vi "simple RX 2955 sync.vi"() -> ()   [LabVIEW 2021]
uses:
  <vilib>/userdefined/High Color/nirio_resource_hc.ctl
  states.ctl
  <vilib>/Analysis/4window.llb/windowTd.ctl
  <vilib>/Analysis/coordinate.llb/Angle Range (Degree).ctl
  <vilib>/Analysis/coordinate.llb/Angle Units.ctl
  <vilib>/Analysis/coordinate.llb/Wrap Angle (scalar).vi
  <instrlib>/_niInstr/DSP/v1/FPGA/Public/Sub VIs/Data Conversion/U32 to IQ - 1 spc - S18.1.vi
  <vilib>/measure/maspectr.llb/FFT Spectrum (Mag-Phase) for 1 Chan (CDB).vi
  <vilib>/FPGAPlugInAG/USRP 2945; 2955/niLvFpga_Open_USRP 2945; 2955.vi
  <vilib>/rvi/interface/common/dynamic/niFpgaDynamicAddResources.vi
  <vilib>/FPGAPlugInAG/Dynamic/niLvFpga_Download_Dynamic.vi
  <vilib>/FPGAPlugInAG/Dynamic/niLvFpga_Run_Dynamic.vi
  <vilib>/rvi/interface/common/niFpgaWaitOnOcc.vi
  <vilib>/Utility/error.llb/Error Cluster From Error Code.vi
  <vilib>/rvi/errors/niLvFpgaAdjustHostInterfaceError.vi
  <vilib>/rvi/interface/nirviOpenFPGA/nirviOpenFPGA.xnode
  FPGA Bitfiles/Streaming 2955 simple.lvbitx
  <vilib>/rvi/interface/nirviMethod/nirviMethod.xnode
  <vilib>/rvi/interface/nirviReadWriteControl/nirviReadWriteControl.xnode
  <instrlib>/niUsrpRio/Config/v1/Host/niUsrpRio Config v1 Host.lvlib
  <vilib>/Analysis/NI_AAL_Angle.lvlib
  <instrlib>/_niInstr/DSP/v1/FPGA/niInstr DSP v1 FPGA.lvlib
  <vilib>/Analysis/NI_AALPro.lvlib
  <vilib>/measure/NI_MAPro.lvlib
  <vilib>/rvi/errors/niLvFpgaMergeErrorWithErrorCode.vi
  <vilib>/rvi/interface/Simulation/niFpgaSimulationCallBeginRW.vi
  <vilib>/FPGAPlugInAG/Dynamic/niLvFpga_ConfigureFifo_Dynamic.vi
  NiFpgaLv.dll
  <vilib>/FPGAPlugInAG/Dynamic/niLvFpga_ReadFifo_Dynamic.vi
panel:
  in  "resource name":T1="USRP_2955"
  in  "computing load":dbl(slide) scale=0.0..20.0
  in  "max queue":i32=20
  out "FPGA lost sampels":u32=262858
  out "dt":dbl=2e-07
  out "delta phase (deg)":dbl[](array[numeric])=[0.0, -114.69647545281569, -168.47745794220134, 21.231862090137405]
  out "scop":dbl[][](graph)
  out "spectrum":cluster{"f0":dbl, "df":dbl, "magnitude":dbl[]}[](graph)
  in  "Number of Elements":u32=2048 step=1024
  in  "reset":bool
  in  "cal phase (deg)":dbl[](array[numeric])=[0.0, 0.0, 0.0, 0.0]
  in  "output sample rate":dbl=5000000.0 format="%#_6pHz"
  in  "frequency shift":dbl=5000000.0 format="%#_6pHz"
  in  "Rx. frequency":dbl=500000000.0 format="%#_6pHz"
  in  "gain":dbl=50.0 min=0.0 max=90.0 step=1.0 format="%#_6pdB"
  # "device"
  # "data out"
  # "Rx params"
  # "RF params"
  # "DSP params"
  # "computing"
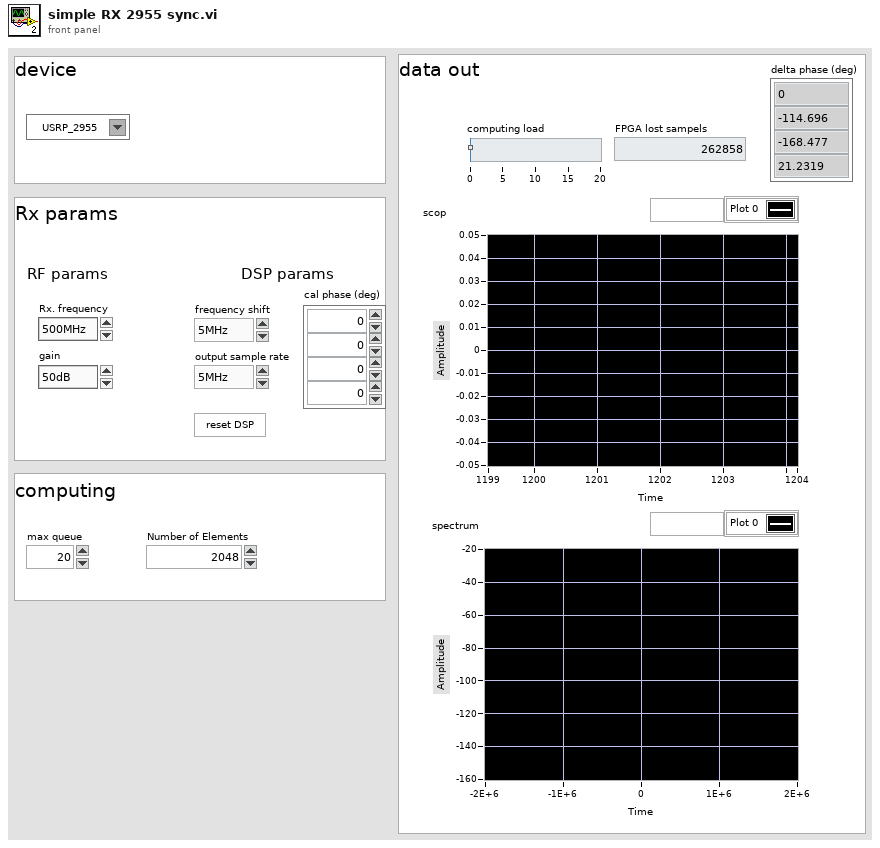
[diagram p1: front panel]
types:
  T1 = typedef "nirio_resource_hc.ctl" = tag
  T2 = typedef "states.ctl" = enum16{"ini", "set basic", "update DSP", "close sesion", "read", "wait"}
  T3 = enum16{"ini", "set basic", "update DSP", "close sesion"}
  T4 = cluster{"daughterboard 0 lo configuration":enum16{"Independent", "Import", "Shared and Export", "Reimport", "Shared"}, "daughterboard 1 lo configuration":enum16{"Independent", "Import", "Shared and Export", "Reimport", "Shared"}}
  T5 = cluster{"output sample rate":fxp<+,48,1>, "delay":fxp<+/-,16,0>, "frequency shift":fxp<+/-,48,0>, "phase":fxp<+/-,21,0>}
  T6 = typedef "niUsrpRio Config v1 Host.lvlib/niUsrpRio Session.ctl" = cluster{"FPGA Interface":refnum<k20>, "RIO Interface Number":u32, "Data Clock Rate":u32, "FPGA Data Clock Rate":u32, "Global Settings Register Bus":T7, "Radio 0 Settings Register Bus":T7, "Radio 1 Settings Register Bus":T7, "Radio Settings Bus Semaphore":T8, "DB Queues":T9[], "Characterization Data Valid?":bool, "EEPROM Header":T10, "Device Data Header":T11, "EEPROM Characterization Header":T12, "Characterization Data":T13[], "FPGA Current Version":u32, "FPGA Oldest Compatible Version":u32, "Fixed Logic Current Version":u32, "Fixed Logic Oldest Compatible Version":u32, "FPGA Radio Settings Bus Current Version":u32, "FPGA Radio Settings Bus Oldest Compatible Version":u32, "FPGA Board Config Current Version":u32, "FPGA Board Config Oldest Compatible Version":u32, "Daughterboard Clock Rate":u32, "daughterboard configuration session handles":u64[]}
  T7 = typedef "niInstr Register Bus v0 Host.lvlib/Register Bus Session.ctl" = refnum<queue>
  T8 = typedef "Semaphore RefNum" = refnum<k1>
  T9 = typedef "niUsrpRio Config v1 Host.lvlib/DB Queue Reference.ctl" = refnum<queue>
  T10 = typedef "niUsrpRio Config v1 Host.lvlib/EEPROM Header.ctl" = cluster{"Checksum":u32, "Product Code":u16, "Hardware Current Version":u16, "Hardware Oldest Compatible Version":u16, "EEPROM Map Current Version":u16, "EEPROM Map Oldest Compatible Version":u16, "User Password":string, "Pointer to Factory Header":u32, "Pointer to User Header":u32, "Recommended Interval":u16, "Number of Reserved Bytes":i32, "Number of Daughterboards":u8, "Daughterboard IDs":u16[], "Daughterboard Serial Numbers":string[]}
  T11 = typedef "niUsrpRio Config v1 Host.lvlib/EEPROM Device Data Header.ctl" = cluster{"Checksum":u32, "Number of Channels":u8, "Number of Gain Settings":u16[], "Pointer to Characterization Data":u32[], "Number of Reserved Bytes":i32, "Number of Frequencies":u16[]}
  T12 = typedef "niUsrpRio Config v1 Host.lvlib/EEPROM Characterization Header.ctl" = cluster{"Checksum":u32, "Date":timestamp, "Temperature":sgl, "Misc. Info":string, "Pointer to Device Data Header":u32, "Number of Reserved Bytes":i32}
  T13 = typedef "niUsrpRio Config v1 Host.lvlib/Characterization Data.ctl" = cluster{"Gains[dB]":dbl[], "Frequencies [Hz]":dbl[], "IQ Imbalance Table":T14[], "Measured Gains[dB]":dbl[][]}
  T14 = typedef "niUsrpRio Config v1 Host.lvlib/IQ Imbalance.ctl" = cluster{"Gain Imbalance [linear]":dbl, "Phase Imbalance [radians]":dbl, "Offset":cdb}
  T15 = cluster{"output sample rate":fxp<+,48,1>, "delay":fxp<+/-,16,0>, "frequency shift":fxp<+/-,48,0>, "phase":fxp<+/-,21,0>}[]
  T16 = typedef "NI_AAL_Angle.lvlib/Angle Units.ctl" = i32
  T17 = typedef "NI_AAL_Angle.lvlib/Angle Range (Degree).ctl" = u16
  T18 = cluster{"dB On (F)":bool, "unwrap phase (F)":bool, "convert to degree (F)":bool}
  T19 = typedef "niInstr DSP v1 Shared.lvlib/IQ Data.ctl" = cluster{"I":fxp<+/-,18,1>, "Q":fxp<+/-,18,1>, "overflow":bool}
  T20 = typedef "NI_AALPro.lvlib/windowTd.ctl" = u32
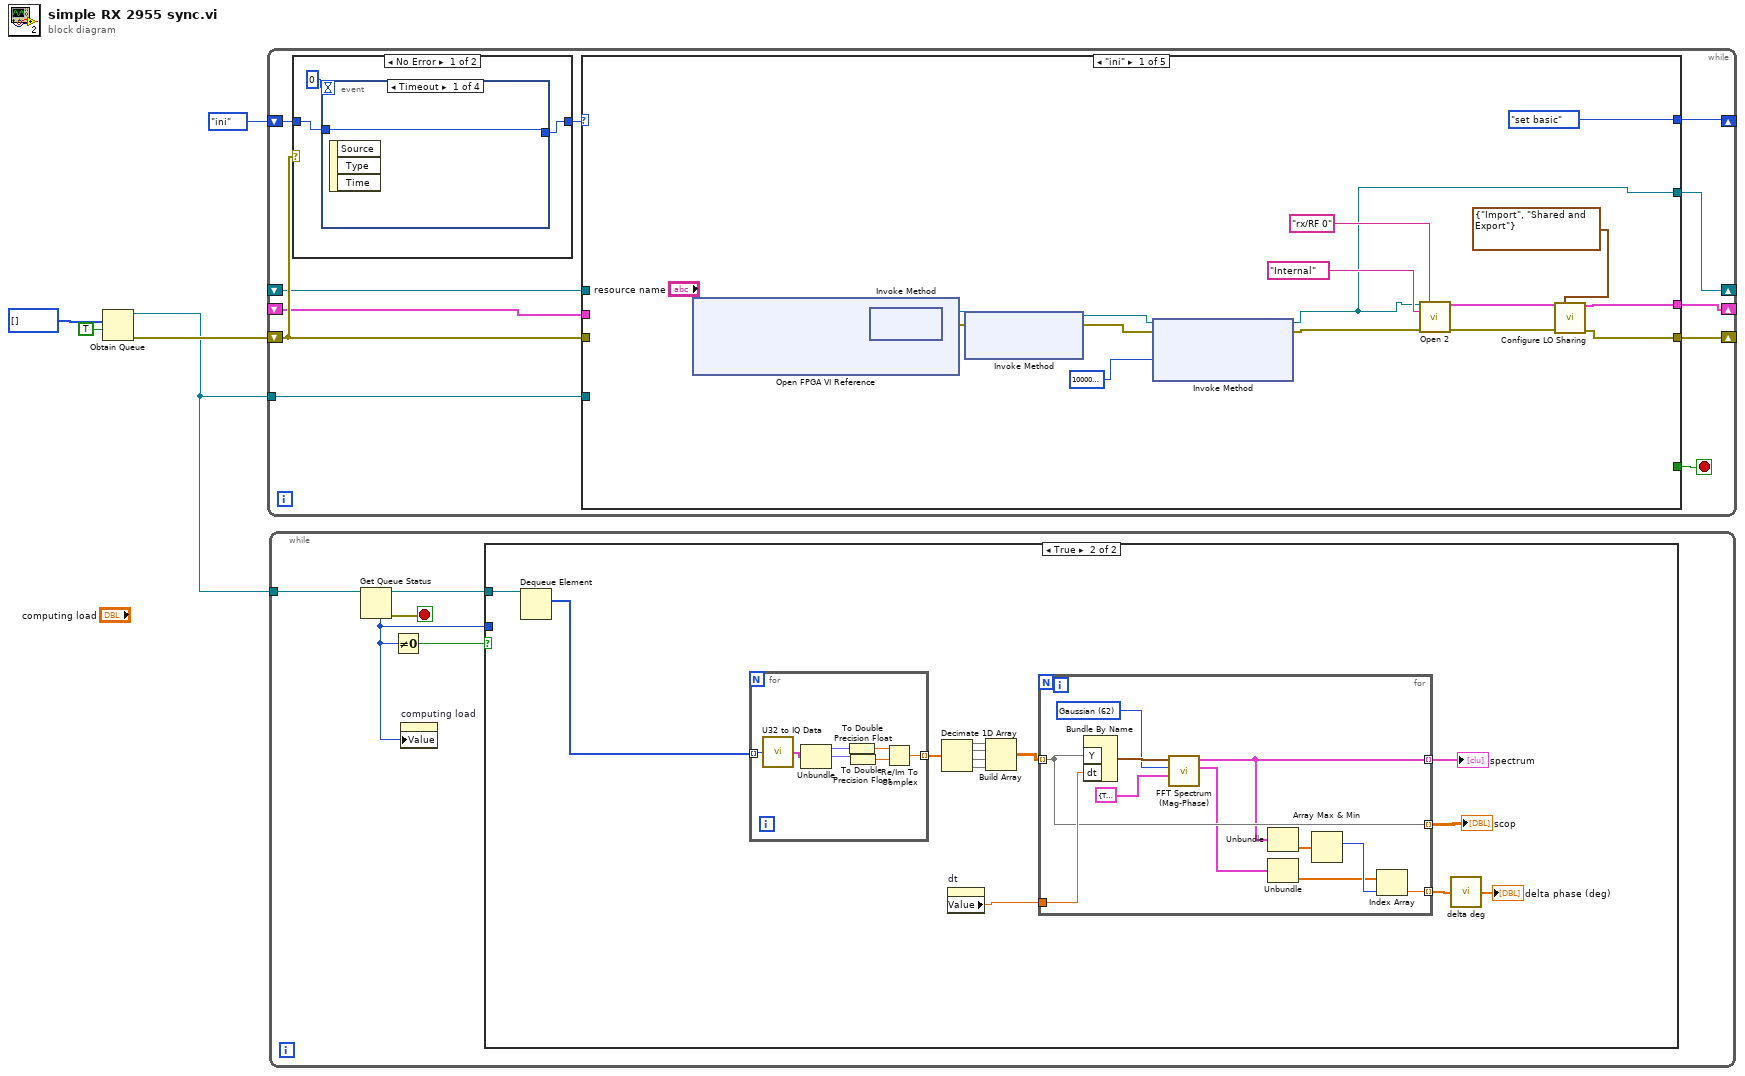
[diagram p0: block diagram]
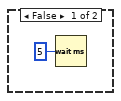
[diagram p2: hidden frame]
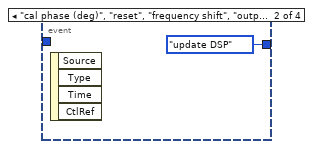
[diagram p3: hidden frame]
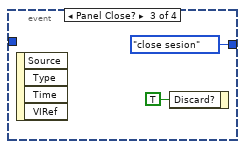
[diagram p4: hidden frame]
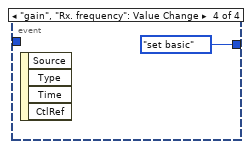
[diagram p5: hidden frame]
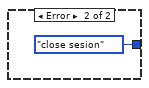
[diagram p6: hidden frame]
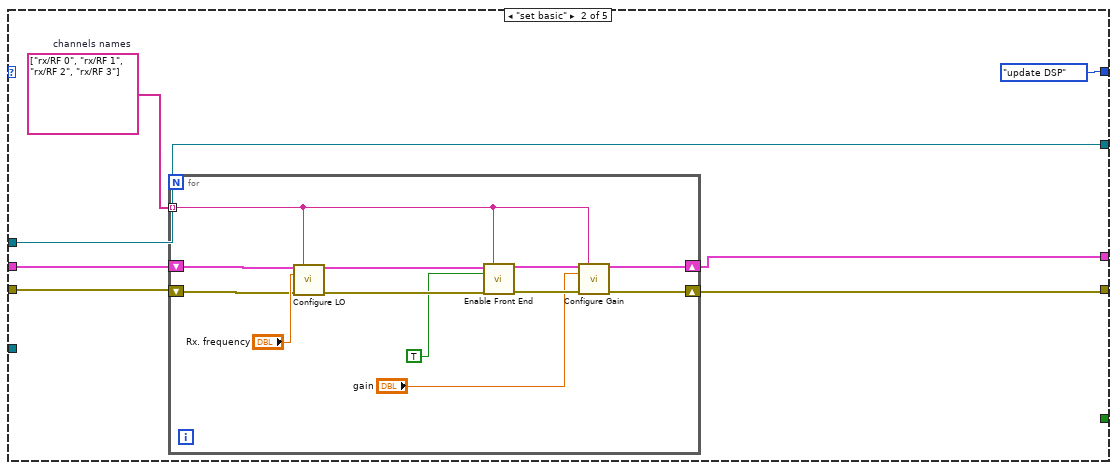
[diagram p7: hidden frame]
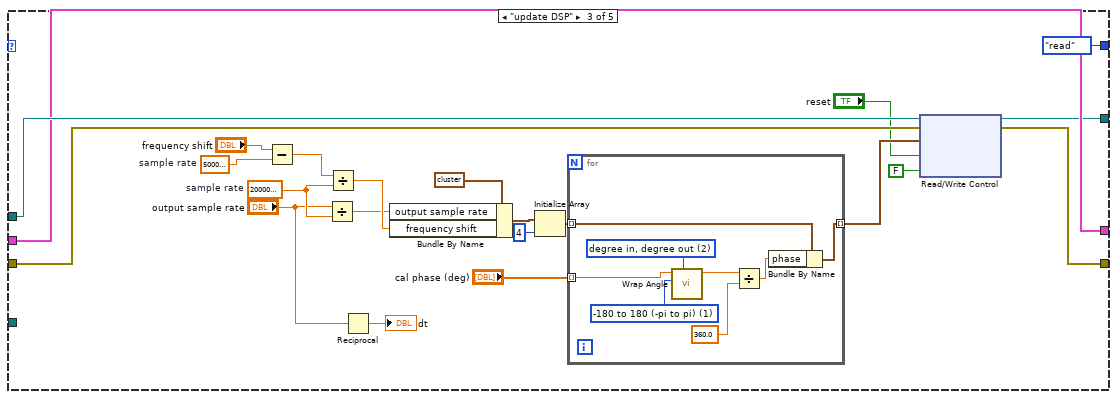
[diagram p8: hidden frame]
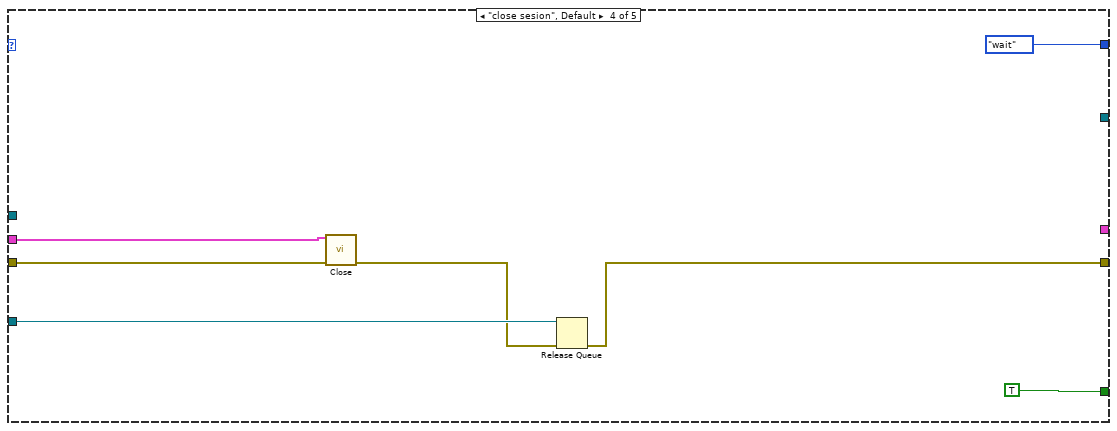
[diagram p9: hidden frame]
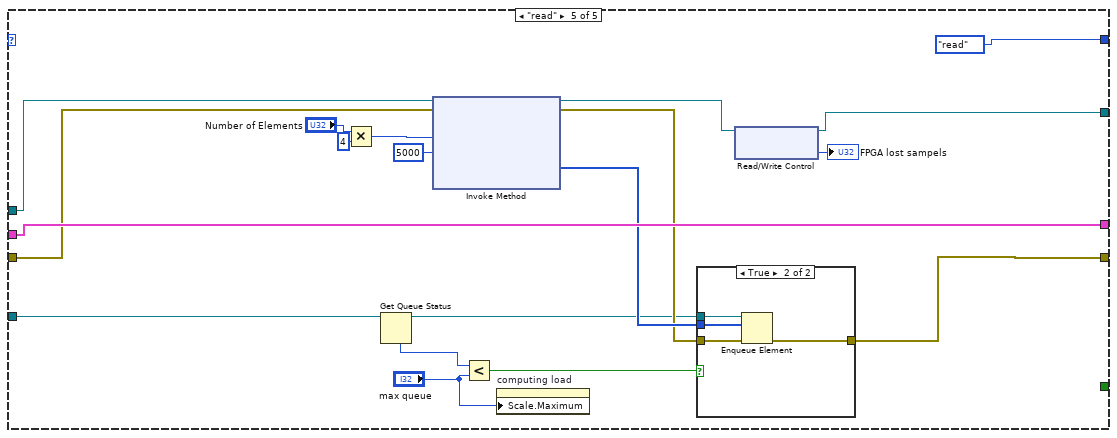
[diagram p10: hidden frame]
diagram:
  n1 = Obtain Queue(element data type=u32[] [] ("Data"), create if not found? (T)=TRUE) -> (queue out=w2:refnum<queue>, error out=w3:errorcluster)  [unwired: 3 in, 1 out]
  n2 = while {
    shift-right: [w8] -> _
    shift-left: states."ini" -> [w16]
    shift-right: [w14] -> _
    shift-left: _ -> [w9]
    shift-right: [w13] -> _
    shift-left: _ -> [w10]
    shift-right: [w12] -> _
    shift-left: w3 -> [w11]
    tunnel: w2 -> [w6]
    stop <- w7 stop-if-true
    n3 = case shown="No Error" w11 {
      tunnel: w16 -> [w18 _]
      tunnel: [w17 T3."close sesion"] -> w15
      frame No Error {
        n4 = event shown="[0] Timeout" {
          selector: _ -> [_ _ _ _]
          dyn-events: _ -> [_ _ _ _]
          timeout: 0 -> [_ _ _ _]
          tunnel: w18 -> [w20 _ _ _]
          tunnel: [w20 states."update DSP" states."close sesion" states."set basic"] -> w17
          event Timeout {
            n5 = event-data() -> ()  [unwired: 1 in, 3 out]
          }
          event "cal phase (deg)", "reset", "frequency shift", "output sample rate": Value Change {
            n6 = event-data() -> ()  [unwired: 1 in, 4 out]
          }
          event Panel Close? {
            n7 = event-data() -> ()  [unwired: 1 in, 4 out]
            n8 = event-data("Discard?"=TRUE) -> ()  [unwired: 1 in, 1 out]
          }
          event "gain", "Rx. frequency": Value Change {
            n9 = event-data() -> ()  [unwired: 1 in, 4 out]
          }
        }
      }
      frame Error {
      }
    }
    n10 = case shown="\"ini\"" w15 {
      tunnel: [w28 w48 w69 _ w105] -> w14
      tunnel: [w34 w46 w71 _ w118] -> w13
      tunnel: [w33 w45 w70 w93 w108] -> w12
      tunnel: w11 -> [_ w50 w72 w99 w111]
      tunnel: w10 -> [_ w49 w71 w98 w118]
      tunnel: w9 -> [_ w48 w73 _ w116]
      tunnel: [states."set basic" states."update DSP" states."read" states."wait" states."read"] -> w8
      tunnel: [_ _ _ TRUE _] -> w7
      tunnel: w6 -> [_ _ _ w95 w104]
      frame "ini" {
        n11 = xnode "Open FPGA VI Reference"("resource name"="resource name") -> ("FPGA VI Reference Out"=w41:refnum<k20>, "error out"=w40:errorcluster)  [unwired: 1 in]
        n12 = xnode "Invoke Method"("FPGA VI Reference In"=w41, "error in"=w40) -> ("FPGA VI Reference Out"=w43:refnum<k20>, "error out"=w42:errorcluster)
        n13 = xnode "Invoke Method"("FPGA VI Reference In"=w43, "error in"=w42) -> ("FPGA VI Reference Out"=w29:refnum<k20>, "error out"=w31:errorcluster)  [unwired: 1 in]
        n14 = xnode "Invoke Method"("FPGA VI Reference In"=w29, "error in"=w31, "Requested Depth"=u32 100000000) -> ("FPGA VI Reference Out"=w28:refnum<k20>, "error out"=w30:errorcluster)  [unwired: 1 out]
        n15 = call <instrlib>:"Open 2.vi"("fpga ref"=w28, "scope"="rx/RF 0", "Reference Frequency Source"="Internal", "error in"=w30) -> ("niUsrpRio Session (out)"=w37:T6, "error out"=w36:errorcluster)  [unwired: 10 in]
        n16 = call "Configure LO Sharing.vi"("niUsrpRio Session in"=w37, "lo config"=T4 {"daughterboard 0 lo configuration"=enum."Import", "daughterboard 1 lo configuration"=enum."Shared and Export"}, "error in"=w36) -> ("niUsrpRio Session out"=w34:T6, "error out"=w33:errorcluster)  [unwired: 11 in]
      }
      frame "set basic" {
        w47 = string[] ["rx/RF 0", "rx/RF 1", "rx/RF 2", "rx/RF 3"]  # channels names
        n17 = for {
          shift-right: [w56] -> w46
          shift-left: w49 -> [w53]
          shift-right: [w55] -> w45
          shift-left: w50 -> [w52]
          tunnel: w47 -> [w51] mode=indexing
          n18 = call <instrlib>:"Configure LO.vi"("niUsrpRio Session"=w53, "scope"=w51, "frequency"="Rx. frequency", "error in"=w52) -> ("niUsrpRio Session (out)"=w62:T6, "error out"=w61:errorcluster)  [unwired: 8 in, 2 out]
          n19 = call <instrlib>:"Enable Front End.vi"("niUsrpRio Session"=w62, "scope"=w51, "enable"=TRUE ("enable 0 2"), "error in"=w61) -> ("niUsrpRio Session (out)"=w60:T6, "error out"=w59:errorcluster)  [unwired: 10 in]
          n20 = call <instrlib>:"Configure Gain.vi"("niUsrpRio Session"=w60, "scope"=w51, "gain"="gain", "error in"=w59) -> ("niUsrpRio Session (out)"=w56:T6, "error out"=w55:errorcluster)  [unwired: 9 in, 1 out]
        }
      }
      frame "update DSP" {
        w77 = 50000000.0  # sample rate
        w80 = 200000000.0  # sample rate
        n21 = Subtract(x="frequency shift", y=w77) -> (x-y=w76:dbl)
        n22 = Divide(x="output sample rate", y=w80) -> (x/y=w79:dbl)
        n23 = Divide(x=w76, y=w80) -> (x/y=w81:dbl)
        n24 = Reciprocal(x="output sample rate") -> (1/x=→"dt":dbl)
        n25 = Bundle By Name(cluster=T5 {"output sample rate"=0.0, "delay"=0.0, "frequency shift"=0.0, "phase"=0.0} ("DSP params"), "output sample rate"=w79, "frequency shift"=w81) -> (w82:T5)
        n26 = Initialize Array(w82, 4 ("dimension size")) -> (w75:T15)
        n27 = for {
          tunnel: w75 -> [w92] mode=indexing
          tunnel: [w91] -> w68 mode=indexing
          tunnel: "cal phase (deg)" -> [w87] mode=indexing
          w85 = T16 2 items=["radian in, radian out", "radian in, degree out", "degree in, degree out", "degree in, radian out"] ("angle units")
          w88 = T17 1 items=["none", "-180 to 180 (-pi to pi)", "0 to 360 (0 to 2pi)"] ("angle range")
          n28 = call-poly <vilib>:"Wrap Angle.vi"("angle units"=w85, "angle range"=w88, "angle in"=w87) -> ("angle out"=w86:dbl)  [unwired: 7 in, 1 out]
          n29 = Divide(x=w86, y=360.0) -> (x/y=w90:dbl)
          n30 = Bundle By Name(cluster=w92, "phase"=w90) -> (w91:T5)
        }
        n31 = xnode "Read/Write Control"("FPGA VI Reference In"=w73, "error in"=w72, "DSP params"=w68, "reset"="reset", "reset"=FALSE) -> ("FPGA VI Reference Out"=w69:refnum<k20>, "error out"=w70:errorcluster)
      }
      frame "close sesion", Default {
        n32 = call <instrlib>:"Close.vi"("niUsrpRio Session"=w98, "error in"=w99) -> ("error out"=w94:errorcluster)  [unwired: 12 in, 1 out]
        n33 = Release Queue(queue=w95, error in (no error)=w94) -> (error out=w93:errorcluster)  [unwired: 1 in, 2 out]
      }
      frame "read" {
        n34 = Multiply(x="Number of Elements", y=u32 4) -> (x*y=w114:u32)
        n35 = Get Queue Status(queue=w104) -> (queue out=w103:refnum<queue>, # elements in queue=w102:i32)  [unwired: 2 in, 6 out]
        n36 = xnode "Invoke Method"("FPGA VI Reference In"=w116, "error in"=w111, "Number of Elements"=w114, "Timeout (ms)"=5000) -> ("FPGA VI Reference Out"=w107:refnum<k20>, "error out"=w109:errorcluster, "Data"=w110:u32[])  [unwired: 1 out]
        n37 = Less?(x=w102, y="max queue") -> (x < y?=w101:bool)
        n38 = property on="computing load" class="Slide (strict)"("Scale.Maximum"="max queue") -> ()  [unwired: 2 in, 2 out]
        n39 = case shown="True" w101 {
          tunnel: w110 -> [_ w123]
          tunnel: w109 -> [w119 w122]
          tunnel: [w119 w121] -> w108
          tunnel: w103 -> [_ w120]
          frame False {
          }
          frame True {
            n40 = Enqueue Element(queue=w120, element=w123, error in (no error)=w122) -> (error out=w121:errorcluster)  [unwired: 1 in, 2 out]
          }
        }
        n41 = xnode "Read/Write Control"("FPGA VI Reference In"=w107) -> ("FPGA VI Reference Out"=w105:refnum<k20>, "lost sampels"=→"FPGA lost sampels":u32)  [unwired: 1 in, 1 out]
      }
    }
  }
  n42 = while {
    tunnel: w2 -> [w128]
    stop <- w125 stop-if-true
    n43 = Get Queue Status(queue=w128) -> (queue out=w126:refnum<queue>, error out=w125:errorcluster, # elements in queue=w124:i32)  [unwired: 2 in, 5 out]
    n44 = Not Equal To 0?(x=w124) -> (x != 0?=w127:bool)
    n45 = property on="computing load" class="Slide (strict)"("Value"=w124) -> ()  [unwired: 2 in, 2 out]
    n46 = case shown="True" w127 {
      tunnel: w124 -> [_ _]
      tunnel: w126 -> [_ w142]
      frame False {
        n47 = Wait (ms)(milliseconds to wait=u32 5) -> ()  [unwired: 1 out]
      }
      frame True {
        n48 = Dequeue Element(queue=w142) -> (element=w141:u32[])  [unwired: 2 in, 3 out]
        n49 = for {
          tunnel: w141 -> [w160] mode=indexing
          tunnel: [w158] -> w140 mode=indexing
          n50 = call-poly <instrlib>:"U32 to IQ Data.vi"("U32 data"=w160) -> ("IQ data"=w159:T19)  [unwired: 14 in]
          n51 = Unbundle(w159) -> ("I"=w157:fxp<+/-,18,1>, "Q"=w156:fxp<+/-,18,1>)  [unwired: 1 out]
          n52 = To Double Precision Float(number=w157) -> (double precision float=w155:dbl)
          n53 = To Double Precision Float(number=w156) -> (double precision float=w154:dbl)
          n54 = Re/Im To Complex(1:w154, 2:w155) -> (0:w158:cdb)
        }
        n55 = Decimate 1D Array(w140) -> (w136:cdb[], w137:cdb[], w138:cdb[], w139:cdb[])
        n56 = property on="dt" class="DigNum (strict)"() -> ("Value"=w132:dbl)  [unwired: 2 in, 2 out]
        n57 = Build Array(w136, w137, w138, w139) -> (w135:cdb[][])
        n58 = for {
          tunnel: w135 -> [w150] mode=indexing
          tunnel: [w148] -> w134 mode=indexing
          tunnel: w132 -> [w152]
          tunnel: [w150] -> w133 mode=indexing
          tunnel: [w143] -> w131 mode=indexing
          w151 = T20 62 items=["Rectangle"=0, "Hanning"=1, "Hamming"=2, "Blackman-Harris"=3, "Exact Blackman"=4, "Blackman"=5, "Flat Top"=6, "4 Term B-Harris "=7, "7 Term B-Harris"=8, "Low Sidelobe"=9, "Blackman Nuttall"=11, "Triangle"=30, "Bartlett-Hanning"=31, "Bohman"=32, "Parzen"=33, "Welch"=34, "Kaiser"=60, "Dolph-Chebyshev"=61, "Gaussian"=62] ("window")
          n59 = Bundle By Name("Y"=w150, "dt"=w152) -> (w153:waveform(cdb))  [unwired: 1 in]
          n60 = call-poly <vilib>:"FFT Spectrum (Mag-Phase).vi"("view"=T18 {"dB On (F)"=TRUE, "unwrap phase (F)"=FALSE, "convert to degree (F)"=TRUE}, "window"=w151, "time signal"=w153) -> ("phase"=w145:cluster{"f0":dbl, "df":dbl, "phase":dbl[]}, "magnitude"=w148:cluster{"f0":dbl, "df":dbl, "magnitude":dbl[]})  [unwired: 4 in, 3 out]
          n61 = Unbundle(w148) -> ("magnitude"=w147:dbl[])  [unwired: 2 out]
          n62 = Unbundle(w145) -> ("phase"=w144:dbl[])  [unwired: 2 out]
          n63 = Array Max & Min(array=w147) -> (max index (indices)=w146:i32)  [unwired: 3 out]
          n64 = Index Array(array=w144, index=w146) -> (element=w143:dbl)
        }
        "spectrum" <- w134
        "scop" <- w133
        n65 = call "delta deg.vi"("array phase"=w131) -> ("delta phase"=→"delta phase (deg)":dbl[])
      }
    }
  }
